vi "8595_driver.vi"(3 "Carrier Freq":string, 7 "error in":errorcluster) -> (13 "error out":errorcluster, 14 "2nd":string, 15 "3rd":string, 16 "4th":string, 17 "Sub":string)   [LabVIEW 2023]
panel:
  out "Sub F":dbl
  out "String 3":string
  out "String":string
  # "SA Acquisition Panel"
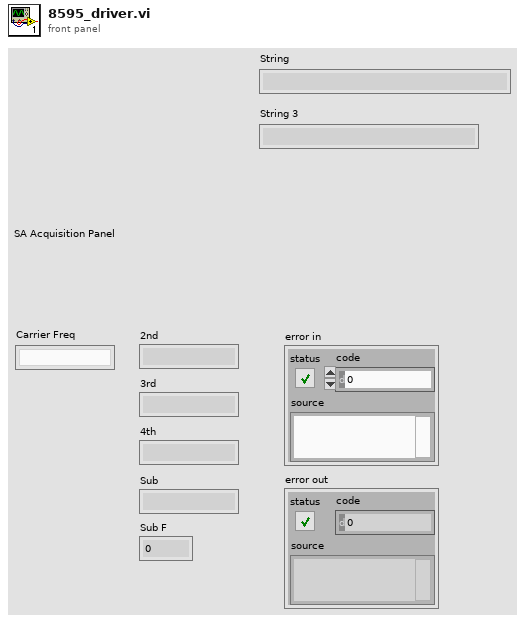
[diagram p1: front panel]
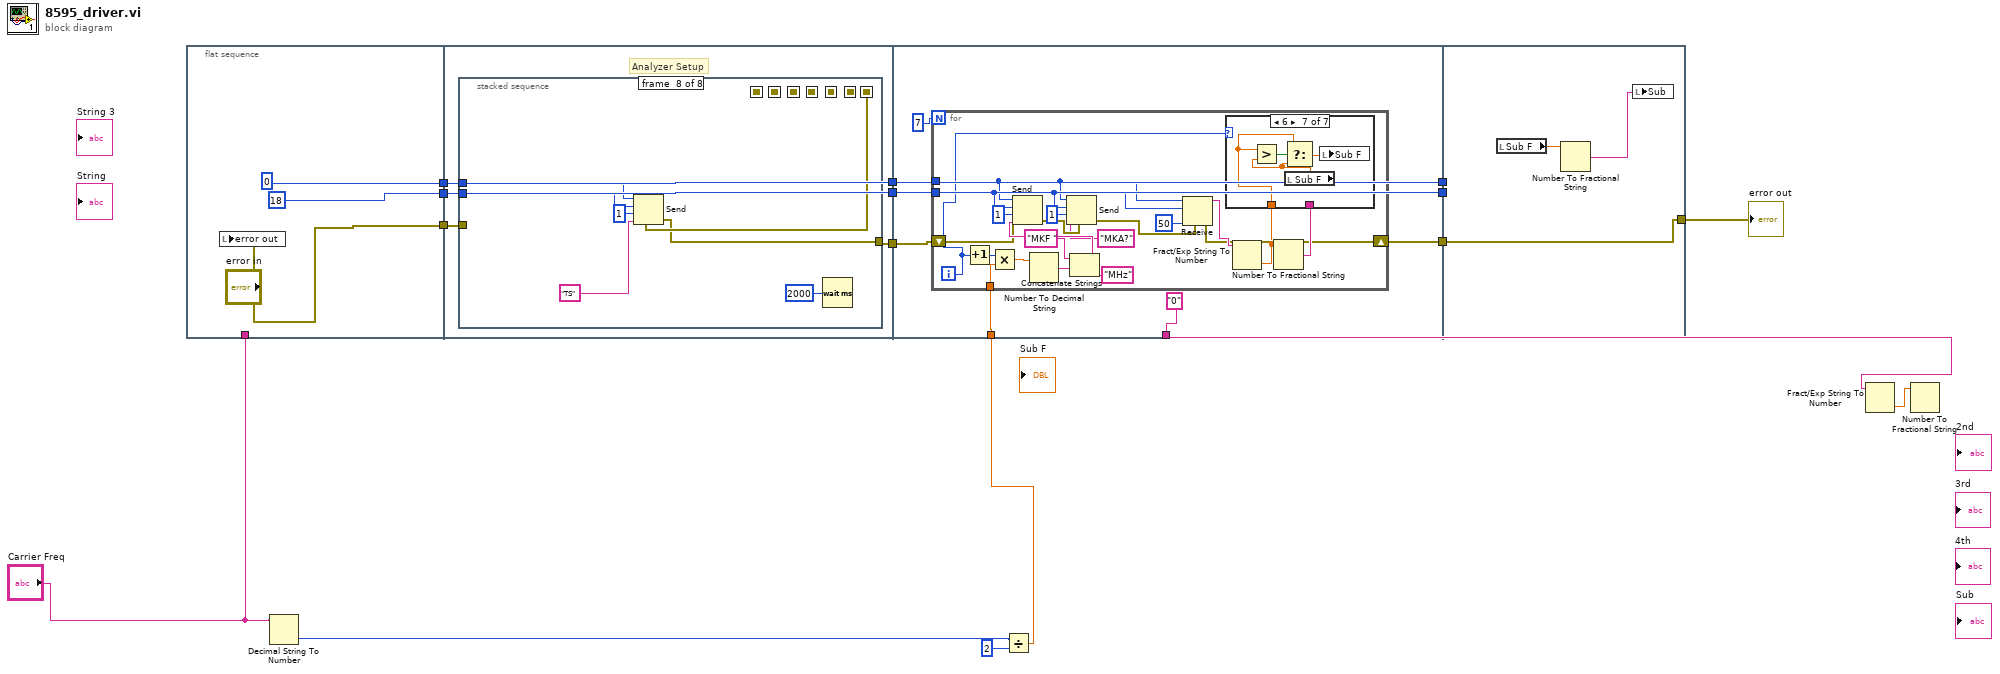
[diagram p0: block diagram]
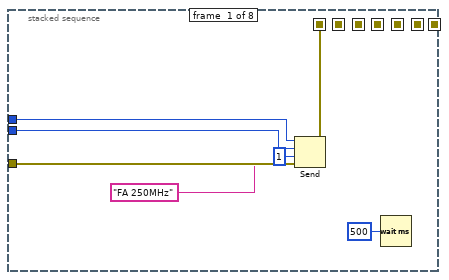
[diagram p2: hidden frame]
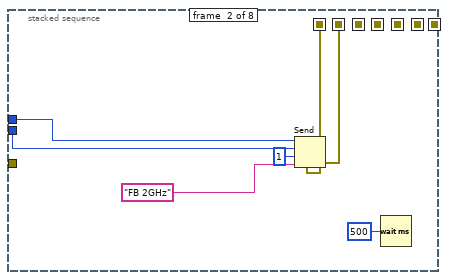
[diagram p3: hidden frame]
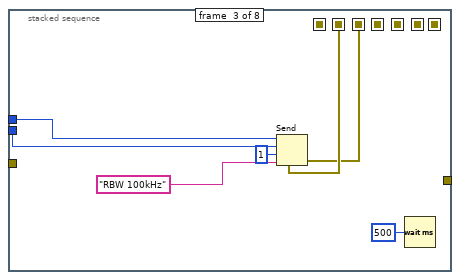
[diagram p4: hidden frame]
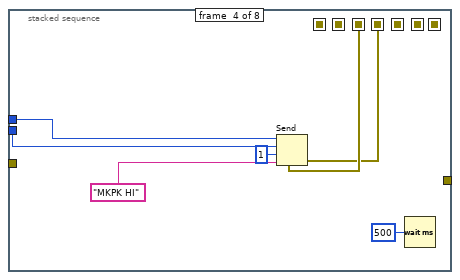
[diagram p5: hidden frame]
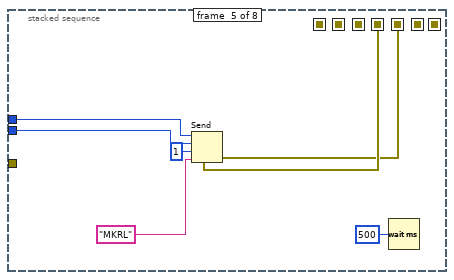
[diagram p6: hidden frame]
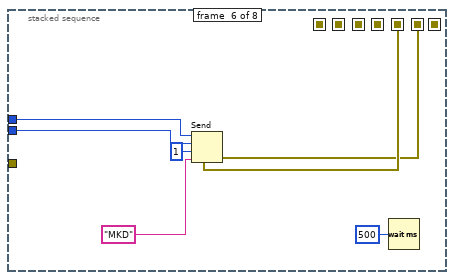
[diagram p7: hidden frame]
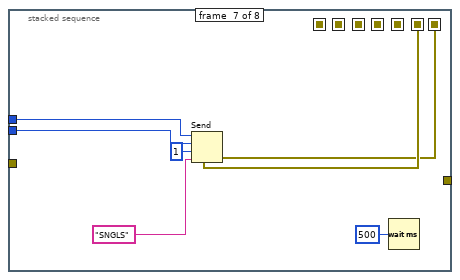
[diagram p8: hidden frame]
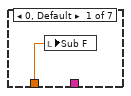
[diagram p9: hidden frame]
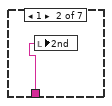
[diagram p10: hidden frame]
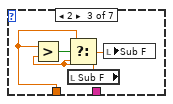
[diagram p11: hidden frame]
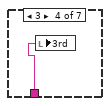
[diagram p12: hidden frame]
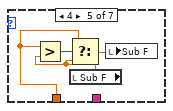
[diagram p13: hidden frame]
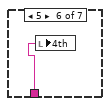
[diagram p14: hidden frame]
diagram:
  n1 = flat-sequence {
    tunnel: "Carrier Freq" -> [_]
    tunnel: ["error in"] -> w11
    tunnel: [0 ("bus")] -> w10
    tunnel: [i16 18 ("address")] -> w9
    tunnel: w11 -> [w23]
    tunnel: w10 -> [w22]
    tunnel: w9 -> [w21]
    tunnel: [w22] -> w8
    tunnel: [w21] -> w7
    tunnel: [w20] -> w6
    tunnel: [w84] -> w16
    tunnel: [w83] -> w15
    tunnel: ["0" ("data string")] -> w13
    tunnel: [w85] -> w14
    tunnel: w8 -> [w84]
    tunnel: w7 -> [w83]
    tunnel: w6 -> [w82]
    tunnel: w1 -> [w81]
    tunnel: w16 -> [_]
    tunnel: w15 -> [_]
    tunnel: w14 -> [w126]
    tunnel: [w126] -> w5
    frame #0 {
      n2 = local write "error out"("error in") -> ()
    }
    frame #1 {
      # "Analyzer Setup"
      n3 = stacked-sequence {
        seq-local: [w26 _ _ _ _ _ _ _] -> [_ w33 _ _ _ _ _ _]
        seq-local: [_ w32 _ _ _ _ _ _] -> [_ _ w40 _ _ _ _ _]
        seq-local: [_ _ w39 _ _ _ _ _] -> [_ _ _ w47 _ _ _ _]
        seq-local: [_ _ _ w46 _ _ _ _] -> [_ _ _ _ w54 _ _ _]
        seq-local: [_ _ _ _ w53 _ _ _] -> [_ _ _ _ _ w61 _ _]
        seq-local: [_ _ _ _ _ w60 _ _] -> [_ _ _ _ _ _ w68 _]
        seq-local: [_ _ _ _ _ _ w66 _] -> [_ _ _ _ _ _ _ w74]
        tunnel: w22 -> [w30 w37 w44 w51 w58 w65 w72 w79]
        tunnel: w21 -> [w29 w36 w43 w50 w57 w64 w71 w78]
        tunnel: w23 -> [w28 _ _ _ _ _ _ _]
        tunnel: [_ _ _ _ _ _ _ w73] -> w20
        frame #0 {
          n4 = Send(0:w30, 2:w29, 3:i16 1 ("mode"), 4:w28, 5:"FA 250MHz" ("string")) -> (8:w26:errorcluster)  [unwired: 2 out]
          n5 = Wait (ms)(milliseconds to wait=u32 500) -> ()  [unwired: 1 out]
        }
        frame #1 {
          n6 = Send(0:w37, 2:w36, 3:i16 1 ("mode"), 4:w33, 5:"FB 2GHz" ("string")) -> (8:w32:errorcluster)  [unwired: 2 out]
          n7 = Wait (ms)(milliseconds to wait=u32 500) -> ()  [unwired: 1 out]
        }
        frame #2 {
          n8 = Send(0:w44, 2:w43, 3:i16 1 ("mode"), 4:w40, 5:"RBW 100kHz" ("string")) -> (8:w39:errorcluster)  [unwired: 2 out]
          n9 = Wait (ms)(milliseconds to wait=u32 500) -> ()  [unwired: 1 out]
        }
        frame #3 {
          n10 = Send(0:w51, 2:w50, 3:i16 1 ("mode"), 4:w47, 5:"MKPK HI" ("string")) -> (8:w46:errorcluster)  [unwired: 2 out]
          n11 = Wait (ms)(milliseconds to wait=u32 500) -> ()  [unwired: 1 out]
        }
        frame #4 {
          n12 = Send(0:w58, 2:w57, 3:i16 1 ("mode"), 4:w54, 5:"MKRL" ("string")) -> (8:w53:errorcluster)  [unwired: 2 out]
          n13 = Wait (ms)(milliseconds to wait=u32 500) -> ()  [unwired: 1 out]
        }
        frame #5 {
          n14 = Send(0:w65, 2:w64, 3:i16 1 ("mode"), 4:w61, 5:"MKD" ("string")) -> (8:w60:errorcluster)  [unwired: 2 out]
          n15 = Wait (ms)(milliseconds to wait=u32 500) -> ()  [unwired: 1 out]
        }
        frame #6 {
          n16 = Send(0:w72, 2:w71, 3:i16 1 ("mode"), 4:w68, 5:"SNGLS" ("string")) -> (8:w66:errorcluster)  [unwired: 2 out]
          n17 = Wait (ms)(milliseconds to wait=u32 500) -> ()  [unwired: 1 out]
        }
        frame #7 {
          n18 = Send(0:w79, 2:w78, 3:i16 1 ("mode"), 4:w74, 5:"TS" ("string")) -> (8:w73:errorcluster)  [unwired: 2 out]
          n19 = Wait (ms)(milliseconds to wait=u32 2000) -> ()  [unwired: 1 out]
        }
      }
    }
    frame #2 {
      n20 = for {
        N: 7 -> [_]
        tunnel: w84 -> [w92]
        tunnel: w83 -> [w91]
        shift-right: [w100] -> w85
        shift-left: w82 -> [w99]
        tunnel: w81 -> [w95]
        i -> [w104]
        n21 = Increment(x=w104) -> (x+1=w97:i32)
        n22 = Multiply(x=w97, y=w95) -> (x*y=w96:dbl)
        n23 = Number To Decimal String(number=w96) -> (decimal integer string=w105:string)  [unwired: 1 in]
        n24 = Concatenate Strings("MKF " ("string"), w105, "MHz" ("string")) -> (w107:string)
        n25 = Send(0:w92, 2:w91, 3:i16 1 ("mode"), 4:w99, 5:w107) -> (8:w93:errorcluster)  [unwired: 2 out]
        n26 = Send(0:w92, 2:w91, 3:i16 1 ("mode"), 4:w93, 5:"MKA?" ("data string")) -> (8:w94:errorcluster)  [unwired: 2 out]
        n27 = Receive(4:w94, 6:50 ("count"), 8:w91, 9:w92) -> (0:w100:errorcluster, 3:w103:string)  [unwired: 1 in, 2 out]
        n28 = Fract/Exp String To Number(string=w103) -> (number=w87:dbl)  [unwired: 3 in, 1 out]
        n29 = Number To Fractional String(number=w87) -> (F-format string=w102:string)  [unwired: 3 in]
        n30 = case shown="6" w104 {
          tunnel: w102 -> [_ w109 _ w114 _ w119 _]
          tunnel: w87 -> [w108 _ w112 _ w115 _ w120]
          frame 0, Default {
            n31 = local write "Sub F"(w108) -> ()
          }
          frame 1 {
            n32 = local write "2nd"(w109) -> ()
          }
          frame 2 {
            n33 = local read "Sub F"() -> (w111:dbl)
            n34 = Greater?(x=w112, y=w111) -> (0:w113:bool)
            n35 = Select(t=w112, s=w113, f=w111) -> (s? t:f=w110:dbl)
            n36 = local write "Sub F"(w110) -> ()
          }
          frame 3 {
            n37 = local write "3rd"(w114) -> ()
          }
          frame 4 {
            n38 = local read "Sub F"() -> (w117:dbl)
            n39 = Greater?(x=w115, y=w117) -> (0:w118:bool)
            n40 = Select(t=w115, s=w118, f=w117) -> (s? t:f=w116:dbl)
            n41 = local write "Sub F"(w116) -> ()
          }
          frame 5 {
            n42 = local write "4th"(w119) -> ()
          }
          frame 6 {
            n43 = local read "Sub F"() -> (w122:dbl)
            n44 = Greater?(x=w120, y=w122) -> (0:w123:bool)
            n45 = Select(t=w120, s=w123, f=w122) -> (s? t:f=w121:dbl)
            n46 = local write "Sub F"(w121) -> ()
          }
        }
      }
    }
    frame #3 {
      n47 = local read "Sub F"() -> (w124:dbl)
      n48 = Number To Fractional String(number=w124) -> (F-format string=w125:string)  [unwired: 3 in]
      n49 = local write "Sub"(w125) -> ()
    }
  }
  n50 = Decimal String To Number(string="Carrier Freq") -> (number=w3:i32)  [unwired: 2 in, 1 out]
  n51 = Divide(x=w3, y=2) -> (x/y=w1:dbl)
  n52 = Fract/Exp String To Number(string=w13) -> (number=w12:dbl)  [unwired: 3 in, 1 out]
  n53 = Number To Fractional String(number=w12) -> ()  [unwired: 3 in, 1 out]
  "error out" <- w5
